vi "Read DMD Calibration Files (SubVI).vi"() -> (1 "DMD2 Int":dbl[][](array[numeric]), 2 "DMD1 Int":dbl[][](array[numeric]), 3 "error out":errorcluster, 4 "DMD1X":dbl[][](array[numeric]), 6 "DMD1Y":dbl[][](array[numeric]), 10 "DMD2X":dbl[][](array[numeric]), 15 "DMD2Y":dbl[][](array[numeric]))   [LabVIEW 2020]
uses:
  <vilib>/Utility/file.llb/Read Delimited Spreadsheet (DBL).vi
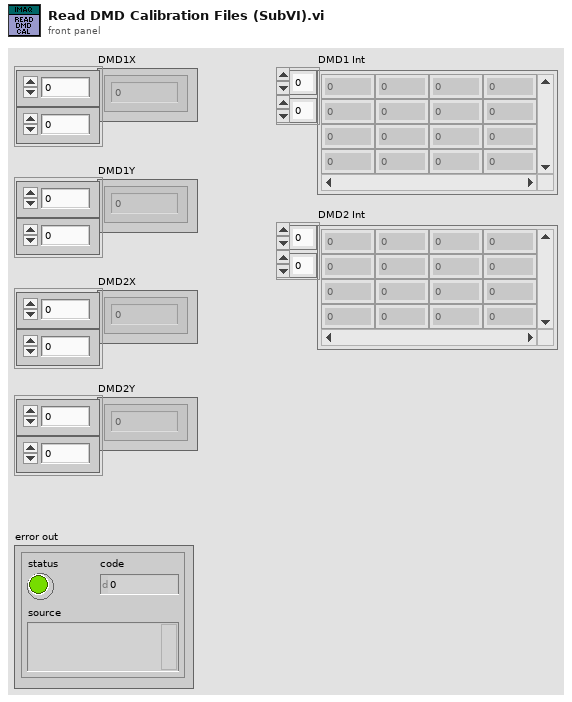
[diagram p1: front panel]
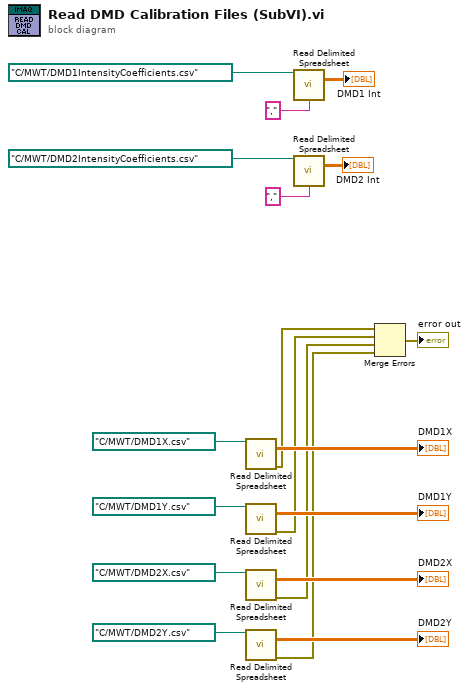
[diagram p0: block diagram]
diagram:
  n1 = call-poly <vilib>:"Read Delimited Spreadsheet.vi"("file path (dialog if empty)"=path "C:/MWT/DMD1X.csv") -> ("all rows"=→"DMD1X":dbl[][], "error out"=w11:errorcluster)  [unwired: 9 in, 4 out]
  n2 = call-poly <vilib>:"Read Delimited Spreadsheet.vi"("file path (dialog if empty)"=path "C:/MWT/DMD1Y.csv") -> ("all rows"=→"DMD1Y":dbl[][], "error out"=w13:errorcluster)  [unwired: 9 in, 4 out]
  n3 = call-poly <vilib>:"Read Delimited Spreadsheet.vi"("file path (dialog if empty)"=path "C:/MWT/DMD2X.csv") -> ("all rows"=→"DMD2X":dbl[][], "error out"=w14:errorcluster)  [unwired: 9 in, 4 out]
  n4 = call-poly <vilib>:"Read Delimited Spreadsheet.vi"("file path (dialog if empty)"=path "C:/MWT/DMD2Y.csv") -> ("all rows"=→"DMD2Y":dbl[][], "error out"=w15:errorcluster)  [unwired: 9 in, 4 out]
  n5 = call-poly <vilib>:"Read Delimited Spreadsheet.vi"("file path (dialog if empty)"=path "C:/MWT/DMD1IntensityCoefficients.csv", "delimiter (\\t)"="," ("delimiter (\\t)")) -> ("all rows"=→"DMD1 Int":dbl[][])  [unwired: 8 in, 5 out]
  n6 = call-poly <vilib>:"Read Delimited Spreadsheet.vi"("file path (dialog if empty)"=path "C:/MWT/DMD2IntensityCoefficients.csv", "delimiter (\\t)"="," ("delimiter (\\t)")) -> ("all rows"=→"DMD2 Int":dbl[][])  [unwired: 8 in, 5 out]
  n7 = Merge Errors(w11, w13, w14, w15) -> (→"error out":errorcluster)
